vi "gestion éclairage face-avant.vi"() -> ()   [LabVIEW 2024]
uses:
  <vilib>/Platform/TimedLoop/XDataNode/timing_clust.ctl
  <vilib>/Platform/TimedLoop/XDataNode/nitl_modes.ctl
  <vilib>/Platform/TimedLoop/XDataNode/wakeup.ctl
  <vilib>/Platform/TimedLoop/XDataNode/XDataNode.xnode
  <vilib>/Platform/TimedLoop/XDataNode/XDNodeRunTimeDep.lvlib
panel:
  out "Orthophoniste":bool
  in  "Couloir":bool caption="OK Button"
  in  "Psy":bool caption="OK Button"
  in  "Ext. Piscine":bool
  in  "Dentiste":bool
  in  "Médecin Kiné":bool
  in  "Orthophoniste\nOstéo":bool
  in  "Couloirs":bool
  in  "Infirmière\nPsy":bool
  in  "Arrêt général":bool
  in  "Secrétariat\nSalle attente":bool
  in  "Jour/nuit":string(combo)
  in  "Simulation présence":bool caption="OK Button"
  in  "Crépuscule":bool caption="OK Button"
  in  "Eclairage total":bool caption="OK Button"
  in  "Horloge":timestamp
  in  "Piscine":bool caption="OK Button"
  in  "Extérieur":bool caption="OK Button"
  in  "Ostéopathe":bool caption="OK Button"
  in  "Dentiste":bool caption="OK Button"
  in  "Orthophoniste":bool caption="OK Button"
  in  "Salle attente":bool caption="OK Button"
  in  "Sécrétariat":bool caption="OK Button"
  in  "Couloir":bool caption="OK Button"
  in  "Salle attente":bool caption="OK Button"
  in  "Infirmière":bool caption="OK Button"
  in  "Kiné":bool caption="OK Button"
  in  "Médecin":bool caption="OK Button"
  out "Dentiste":bool
  out "Piscine 2":bool
  out "Piscine 1":bool
  out "Ext. 2":bool
  out "Ext. 1":bool
  out "Attente 0":bool
  out "Secrétariat":bool
  out "Couloir 0":bool
  out "Ostéopathe":bool
  out "Attente 1":bool
  out "Psychologue":bool
  out "Couloir 2":bool
  out "Couloir 1":bool
  out "Infirmière":bool
  out "Kinésithérapeute":bool
  out "Médecin":bool
  # "GESTION AUTOMATISEE DE L'ECLAIRAGE D'UNE MAISON MEDICALE"
  # "ETAGE"
  # "REZ-DE-CHAUSSEE"
  # "COMMANDES"
  # "Etage"
  # "Modes"
  # "Rez-de-Chaussée"
  # "DISJONCTEURS"
  # "Extérieur"
  # "Horloge"
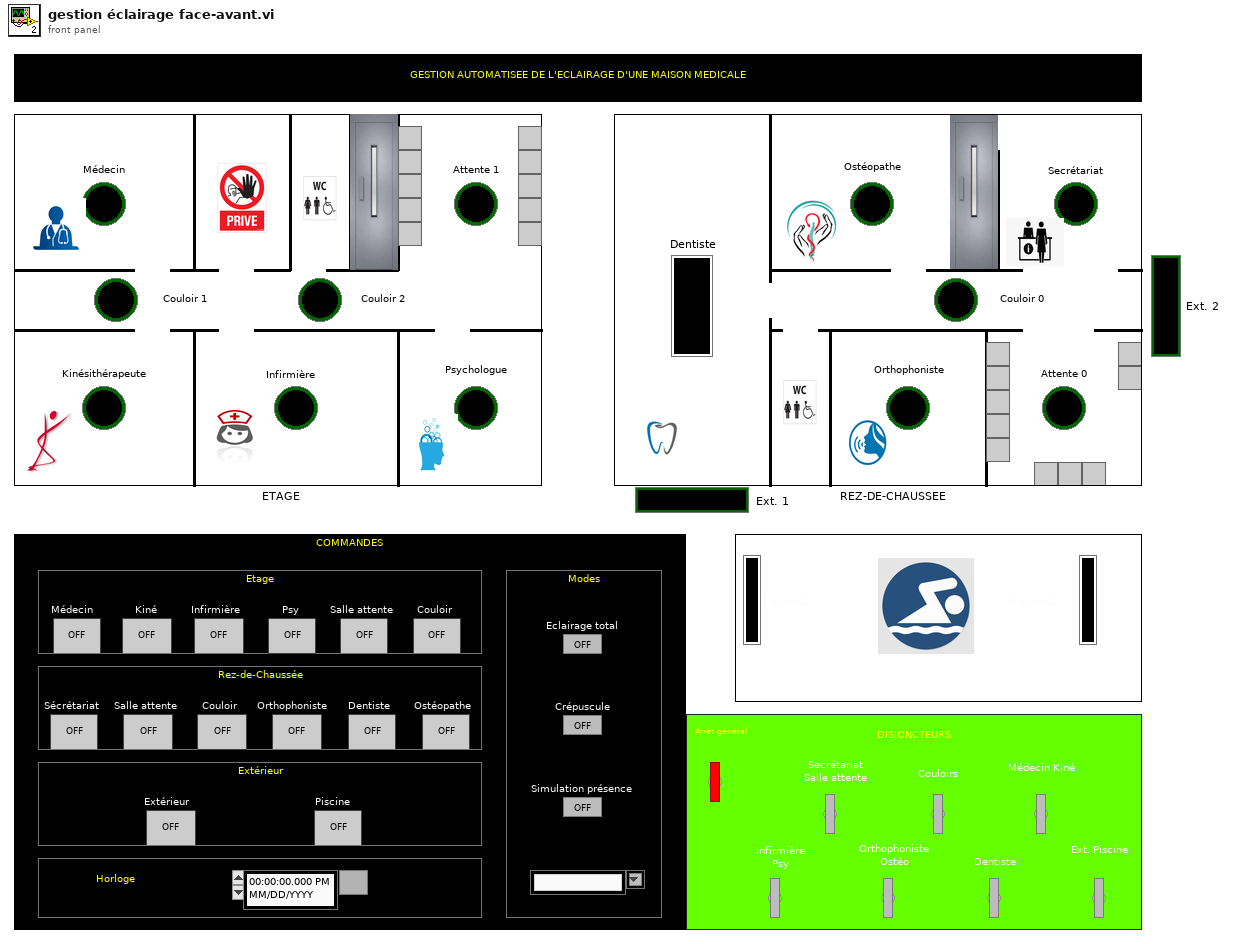
[diagram p1: front panel]
types:
  T1 = typedef "XDNodeRunTimeDep.lvlib/timing_clust.ctl" = cluster{"Expected End [f-1]":u64, "Actual End [f-1]":u64, "Finished Late? [f-1]":bool, "Expected End [i-1]":u64, "Actual End [i-1]":u64, "Finished Late? [i-1]":bool, "Expected Start [i]":u64, "Actual Start [i]":u64, "Expected Start [f]":u64, "Actual Start [f]":u64, "Source Name":string, "Structure Name":string, "Period":i64, "Deadline":i64, "Offset":i64, "Start":i64, "Priority":i32, "Timeout":i32, "Mode":T2, "Wakeup Reason":T3, "Error":errorcluster, "Source Type":string, "Secondary Source Type":string, "Global End Time":u64, "Global Start Time":u64, "Frame Duration":u64, "Iteration Duration":u64, "Assigned CPU":i32, "I/O Scan Engine Mode":u32}
  T2 = typedef "XDNodeRunTimeDep.lvlib/nitl_modes.ctl" = enum32{"No Change", "Process missed periods, maintain original phase", "Discard missed periods, maintain original phase", "Process missed periods, ignore original phase", "Discard missed periods, ignore original phase"}
  T3 = typedef "XDNodeRunTimeDep.lvlib/wakeup.ctl" = enum32{"Normal", "Aborted", "Asynchronous wakeup", "Timing source error", "Timed loop error", "Timeout"}
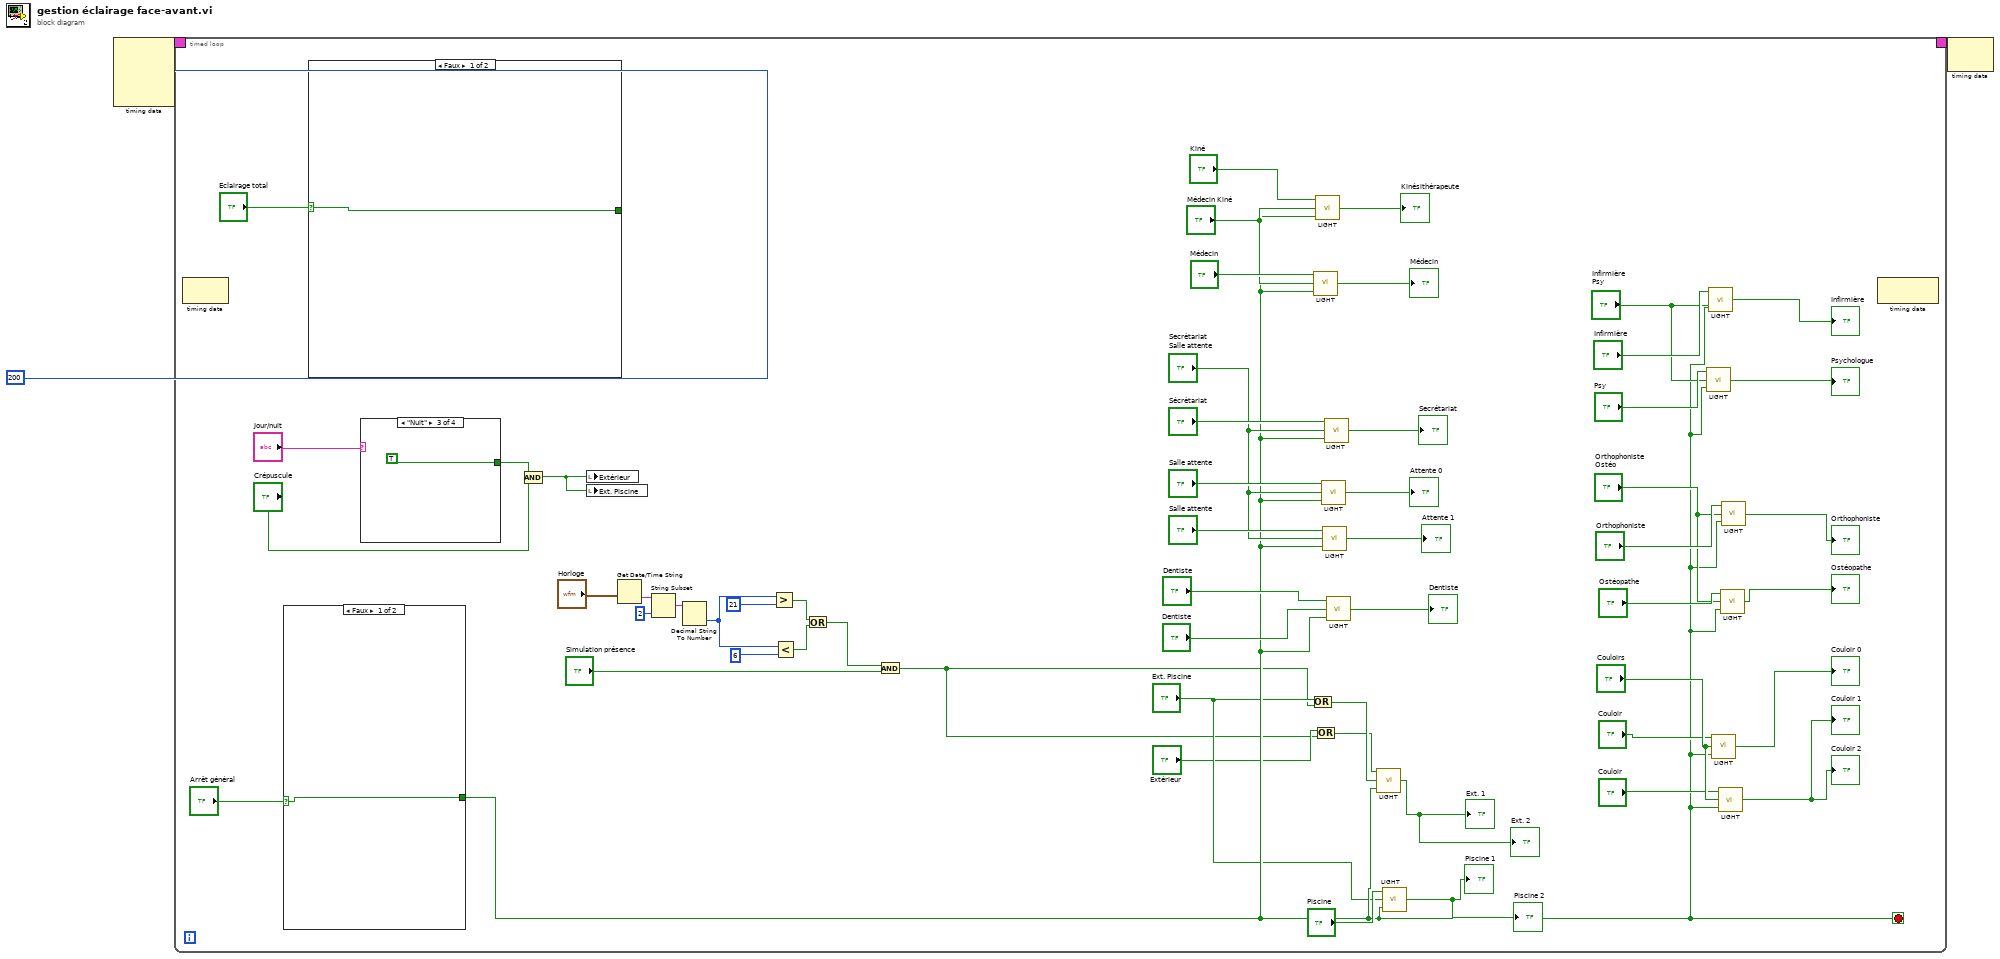
[diagram p0: block diagram]
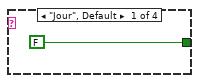
[diagram p2: hidden frame]
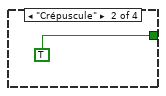
[diagram p3: hidden frame]
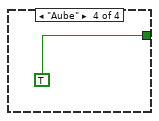
[diagram p4: hidden frame]
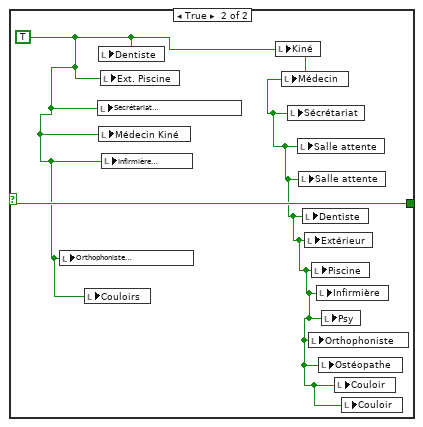
[diagram p5: hidden frame]
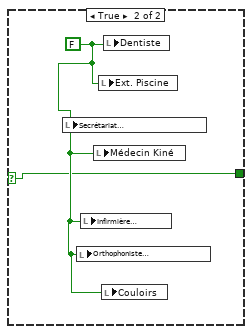
[diagram p6: hidden frame]
diagram:
  n1 = node-c288(i64 200 ("Période")) -> (w3:T1)  [unwired: 3 in]
  n2 = timed-loop {
    timing: w3 -> [_]
    timing-out: [_] -> w2
    stop <- w26 stop-if-true
    n3 = node-c288() -> ()  [unwired: 1 in, 1 out]
    n4 = case shown="Faux" "Arrêt général" {
      selector: "Arrêt général" -> [w67 w68]
      tunnel: [w67 w68] -> w26
      frame False {
      }
      frame True {
        w69 = FALSE
        n5 = local write "Secrétariat\nSalle attente"(w69) -> ()
        n6 = local write "Orthophoniste\nOstéo"(w69) -> ()
        n7 = local write "Infirmière\nPsy"(w69) -> ()
        n8 = local write "Médecin Kiné"(w69) -> ()
        n9 = local write "Ext. Piscine"(w69) -> ()
        n10 = local write "Couloirs"(w69) -> ()
        n11 = local write "Dentiste"(w69) -> ()
      }
    }
    n12 = case shown="Faux" "Eclairage total" {
      selector: "Eclairage total" -> [w64 w66]
      tunnel: [w64 w66] -> _
      frame False {
      }
      frame True {
        w65 = TRUE
        n13 = local write "Orthophoniste\nOstéo"(w65) -> ()
        n14 = local write "Couloirs"(w65) -> ()
        n15 = local write "Secrétariat\nSalle attente"(w65) -> ()
        n16 = local write "Dentiste"(w65) -> ()
        n17 = local write "Médecin Kiné"(w65) -> ()
        n18 = local write "Ext. Piscine"(w65) -> ()
        n19 = local write "Infirmière\nPsy"(w65) -> ()
        n20 = local write "Kiné"(w65) -> ()
        n21 = local write "Médecin"(w65) -> ()
        n22 = local write "Sécrétariat"(w65) -> ()
        n23 = local write "Salle attente"(w65) -> ()
        n24 = local write "Salle attente"(w65) -> ()
        n25 = local write "Dentiste"(w65) -> ()
        n26 = local write "Extérieur"(w65) -> ()
        n27 = local write "Orthophoniste"(w65) -> ()
        n28 = local write "Piscine"(w65) -> ()
        n29 = local write "Infirmière"(w65) -> ()
        n30 = local write "Ostéopathe"(w65) -> ()
        n31 = local write "Psy"(w65) -> ()
        n32 = local write "Couloir"(w65) -> ()
        n33 = local write "Couloir"(w65) -> ()
      }
    }
    n34 = case shown="\"Nuit\"" "Jour/nuit" {
      tunnel: [FALSE TRUE TRUE TRUE] -> w21
      frame "Jour", Default {
      }
      frame "Crépuscule" {
      }
      frame "Nuit" {
      }
      frame "Aube" {
      }
    }
    n35 = And(x=w21, y="Crépuscule") -> (x .and. y?=w20:bool)
    n36 = local write "Extérieur"(w20) -> ()
    n37 = local write "Ext. Piscine"(w20) -> ()
    n38 = Get Date/Time String(seconds (now)="Horloge") -> (time string=w18:string)  [unwired: 2 in, 1 out]
    n39 = String Subset(string=w18, length (rest)=2 ("longueur (reste)")) -> (substring=w16:string)  [unwired: 1 in]
    n40 = Decimal String To Number(string=w16) -> (number=w12:i32)  [unwired: 2 in, 1 out]
    n41 = Greater?(x=w12, y=21) -> (0:w14:bool)
    n42 = Less?(x=w12, y=6) -> (x < y?=w15:bool)
    n43 = Or(x=w14, y=w15) -> (x .or. y?=w9:bool)
    n44 = And(x=w9, y="Simulation présence") -> (x .and. y?=w6:bool)
    n45 = Or(x="Ext. Piscine", y=w6) -> (x .or. y?=w5:bool)
    n46 = call "LIGHT.vi"("Disjoncteur general"=w26, "Disjonct"="Médecin Kiné", "Interrupteur"="Médecin") -> ("LED"=→"Médecin":bool)
    n47 = Or(x="Extérieur", y=w6) -> (x .or. y?=w4:bool)
    n48 = call "LIGHT.vi"("Disjoncteur general"=w26, "Disjonct"="Médecin Kiné", "Interrupteur"="Kiné") -> ("LED"=→"Kinésithérapeute":bool)
    n49 = call "LIGHT.vi"("Disjoncteur general"=w26, "Disjonct"="Secrétariat\nSalle attente", "Interrupteur"="Salle attente") -> ("LED"=→"Attente 0":bool)
    n50 = call "LIGHT.vi"("Disjoncteur general"=w26, "Disjonct"="Secrétariat\nSalle attente", "Interrupteur"="Salle attente") -> ("LED"=→"Attente 1":bool)
    n51 = call "LIGHT.vi"("Disjoncteur general"=w26, "Disjonct"="Secrétariat\nSalle attente", "Interrupteur"="Sécrétariat") -> ("LED"=→"Secrétariat":bool)
    n52 = call "LIGHT.vi"("Disjoncteur general"=w26, "Disjonct"="Dentiste", "Interrupteur"="Dentiste") -> ("LED"=→"Dentiste":bool)
    n53 = call "LIGHT.vi"("Disjoncteur general"=w26, "Disjonct"=w5, "Interrupteur"=w4) -> ("LED"=→"Ext. 1" →"Ext. 2":bool)
    n54 = call "LIGHT.vi"("Disjoncteur general"=w26, "Disjonct"="Ext. Piscine", "Interrupteur"="Piscine") -> ("LED"=→"Piscine 1" →"Piscine 2":bool)
    n55 = call "LIGHT.vi"("Disjoncteur general"=w26, "Disjonct"="Infirmière\nPsy", "Interrupteur"="Psy") -> ("LED"=→"Psychologue":bool)
    n56 = call "LIGHT.vi"("Disjoncteur general"=w26, "Disjonct"="Infirmière\nPsy", "Interrupteur"="Infirmière") -> ("LED"=→"Infirmière":bool)
    n57 = call "LIGHT.vi"("Disjoncteur general"=w26, "Disjonct"="Couloirs", "Interrupteur"="Couloir") -> ("LED"=→"Couloir 0":bool)
    n58 = call "LIGHT.vi"("Disjoncteur general"=w26, "Disjonct"="Couloirs", "Interrupteur"="Couloir") -> ("LED"=→"Couloir 1" →"Couloir 2":bool)
    n59 = call "LIGHT.vi"("Disjoncteur general"=w26, "Disjonct"="Orthophoniste\nOstéo", "Interrupteur"="Ostéopathe") -> ("LED"=→"Ostéopathe":bool)
    n60 = call "LIGHT.vi"("Disjoncteur general"=w26, "Disjonct"="Orthophoniste\nOstéo", "Interrupteur"="Orthophoniste") -> ("LED"=→"Orthophoniste":bool)
    n61 = node-c288() -> ()  [unwired: 1 in, 1 out]
  }
  n62 = node-c288(w2) -> ()  [unwired: 1 out]
